vi "Deliver Request.vi"(8 "error in (no error)":errorcluster, 10 "Request":refnum<class "request.lvclass">, 11 "output_poller_actor in":refnum<class "output_poller_actor.lvclass">) -> (0 "error out":errorcluster, 3 "output_poller_actor out":refnum<class "output_poller_actor.lvclass">)   [LabVIEW 2015, in "output_poller_actor.lvclass"]
uses:
  output_poller_actor.lvclass
  Request/request.lvclass
  output_poller_actor.lvclass/output_poller_actor.ctl
  Output Actor Messages/Do Request Msg/Do Request Msg.lvclass/Do Request Msg.ctl
  <vilib>/ActorFramework/Message Enqueuer/Message Enqueuer.lvclass/Message Enqueuer.ctl
  <vilib>/ActorFramework/Message Enqueuer/Enqueue.vi
  <vilib>/ActorFramework/Message Priority Queue/Priority Enqueue.vi
  Output Actor Messages/Do Request Msg/Do Request Msg.lvclass
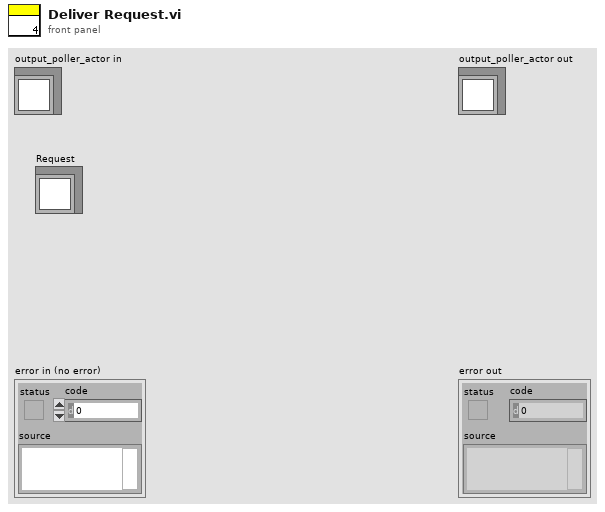
[diagram p1: front panel]
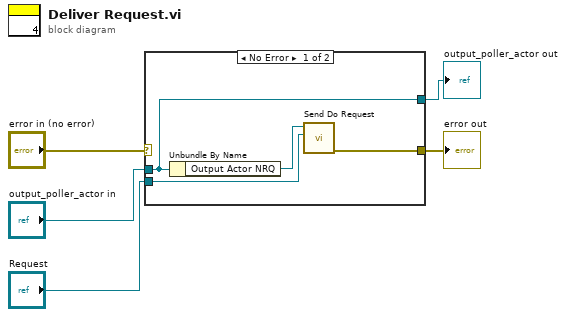
[diagram p0: block diagram]
diagram:
  n1 = case shown="No Error" "error in (no error)" {
    selector: "error in (no error)" -> [_ w10]
    tunnel: [w7 w10] -> w5
    tunnel: [w6 w11] -> w4
    tunnel: "Request" -> [w8 _]
    tunnel: "output_poller_actor in" -> [w6 w11]
    frame No Error {
      n2 = Unbundle By Name(w6) -> ("Output Actor NRQ"=w9:refnum<class "Message Enqueuer.lvclass">)
      n3 = call "Send Do Request.vi"("request.lvclass"=w8, "Message Enqueuer"=w9) -> ("error out"=w7:errorcluster)  [unwired: 8 in, 1 out]
    }
    frame Error {
    }
  }
  "error out" <- w5
  "output_poller_actor out" <- w4
